vi "Caps_GUI.vi"(11 "GUI_cluster":T1={"Sub Panel"=refnum, "GUIdevice"="Bella_LP_Mode", "CtlRef"=refnum, "User Event in"=refnum}) -> ()   [LabVIEW 2013]
uses:
  Shared/GUI_Template/GUI_master/tcp_new_data_event.ctl
  Shared/GUI_Template/GUI_master/tcp new data cluster.ctl
  Controls/GUI_cluster.ctl
  Controls/eventtypdef1.ctl
panel:
  out "GUIdevice 6":string="Bella_LP_Mode"
  out "GUIdevice 5":string="Bella_LP_Mode"
  out "GUIdevice 4":string="Bella_LP_Mode"
  out "GUIdevice 3":string="Bella_LP_Mode"
  out "GUIdevice 2":string="Bella_LP_Mode"
  out "timing (ns) 2":dbl
  in  "timing (ns)":dbl
  out "pressureCap1::6":dbl caption="pressure read" min=0.0 max=10.0
  out "pressureCap2::6":dbl caption="pressure read" min=0.0 max=10.0
  in  "pressure::5":dbl caption="pressure" min=0.0 max=200.0
  in  "pressure::4":dbl caption="pressure" min=0.0 max=200.0
  in  "discharge2::3":bool caption="Trigger"
  in  "discharge1::3":bool caption="Trigger"
  out "AI_mean.Channel 3::2":dbl caption="read \nvoltage" min=0.0 max=0.0
  in  "voltage.hv 2::1":dbl caption="set \nvoltage" min=0.0 max=30.0
  out "AI_mean.Channel 0::2":dbl caption="read \nvoltage" min=0.0 max=0.0
  in  "voltage.hv 1::1":dbl caption="set \nvoltage" min=0.0 max=30.0
  out "tcp data event":T2
  out "GUIdevice 1":string="Bella_LP_Mode"
  in  "stop":bool
  # "CAP2"
  # "CAP1"
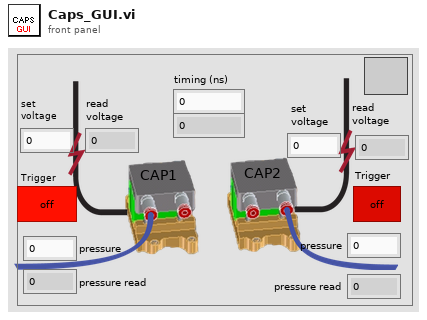
[diagram p1: front panel]
types:
  T1 = typedef "GUI_cluster.ctl" = cluster{"Sub Panel":refnum<vi>, "GUIdevice":string, "CtlRef":refnum<vi>, "User Event in":refnum<user-event>}
  T2 = typedef "tcp_new_data_event.ctl" = refnum<user-event>
  T3 = typedef "eventtypdef1.ctl" = cluster{"label":string, "Sub Panel":refnum<vi>, "CtlRef":refnum<vi>, "This VI":refnum<vi>}
  T4 = typedef "tcp new data cluster.ctl" = cluster{"EventEnum":enum16{"new data", "connection status update"}, "Device name":string}
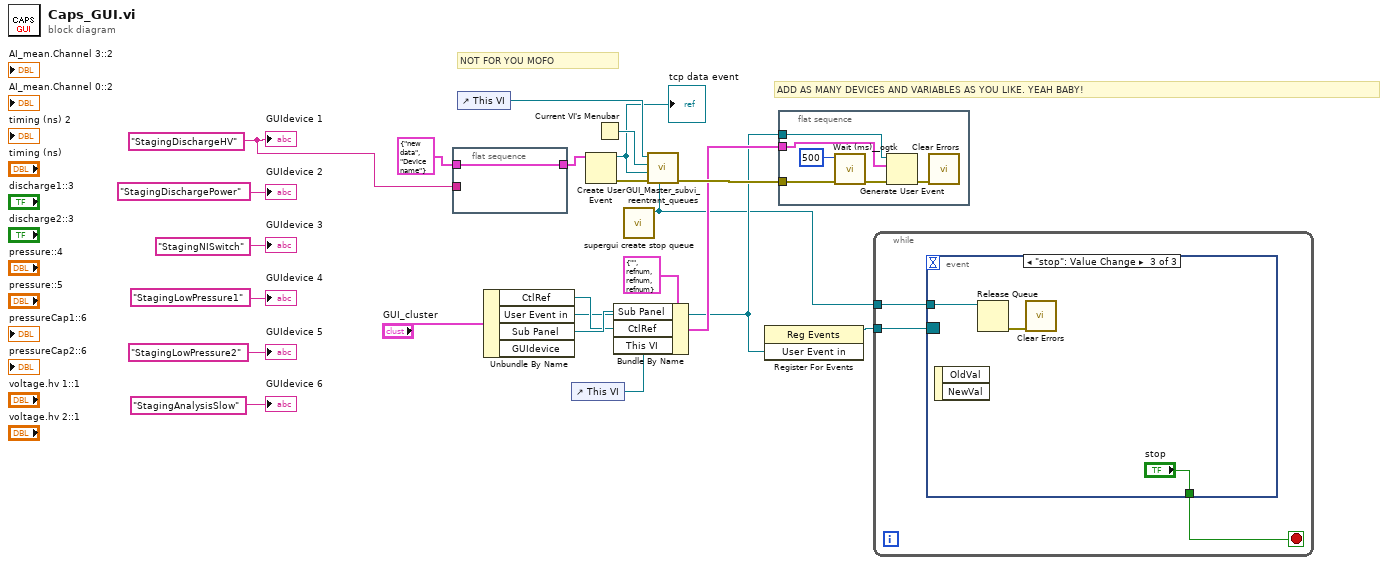
[diagram p0: block diagram]
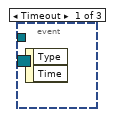
[diagram p2: hidden frame]
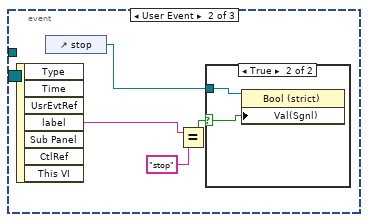
[diagram p3: hidden frame]
diagram:
  w2 = "StagingDischargeHV" ("GUIdevice 23")
  # "ADD AS MANY DEVICES AND VARIABLES AS YOU LIKE. YEAH BABY!"
  # "NOT FOR YOU MOFO"
  n1 = flat-sequence {
    tunnel: T4 {"EventEnum"=enum."new data", "Device name"="Device name"} ("New Event") -> [w23]
    tunnel: w2 -> [_]
    tunnel: [w23] -> w1
    frame #0 {
    }
  }
  n2 = control-ref of="This VI"() -> (w22:refnum<vi>)
  n3 = Unbundle By Name("GUI_cluster") -> ("CtlRef"=w15:refnum<vi>, "User Event in"=w5:refnum<user-event>, "Sub Panel"=w16:refnum<vi>)  [unwired: 1 out]
  n4 = control-ref of="This VI"() -> (w14:refnum<vi>)
  n5 = Create User Event(user event datatype=w1) -> (user event=w19:refnum<user-event>, error out=w20:errorcluster)  [unwired: 1 in]
  "tcp data event" <- w19
  n6 = Current VI's Menubar() -> (w21:refnum<k9>)
  n7 = Bundle By Name(cluster=T3 {"label"="", "Sub Panel"=refnum, "CtlRef"=refnum, "This VI"=refnum} ("event data"), "Sub Panel"=w16, "CtlRef"=w15, "This VI"=w14) -> (w12:T3)
  n8 = call "supergui create stop queue.vi"() -> ("STOP Queue out"=w4:refnum<queue>)  [unwired: 11 in]
  n9 = call "GUI_Master_subvi_reentrant_queues.vi"("STOP Queue in"=w4, "error in (no error)"=w20, "tcp data event"=w19, "Caller menu reference"=w21, "Caller VI ref"=w22) -> ("error out"=w13:errorcluster)  [unwired: 6 in]
  n10 = register-events(w5) -> (reference out=w6:refnum<event-registration>)  [unwired: 2 in, 1 out]
  n11 = flat-sequence {
    tunnel: w13 -> [w26]
    tunnel: w5 -> [w29]
    tunnel: w12 -> [w28]
    frame #0 {
      n12 = call <userlib>:"Wait (ms)__ogtk.vi"("error in (no error)"=w26, "milliseconds to wait"=u32 500) -> ("error out"=w25:errorcluster)  [unwired: 8 in, 1 out]
      n13 = Generate User Event(user event=w29, event data cluster=w28, error in=w25) -> (error out=w27:errorcluster)  [unwired: 1 in, 1 out]
      n14 = call <vilib>:"Clear Errors.vi"("error in (no error)"=w27) -> ()  [unwired: 6 in, 1 out]
    }
  }
  n15 = while {
    tunnel: w6 -> [w32]
    tunnel: w4 -> [w30]
    stop <- w31 stop-if-true
    n16 = event shown="[2] \"stop\": Value Change" {
      selector: w32 -> [_ _ _]
      dyn-events: _ -> [_ _ _]
      timeout: _ -> [_ _ _]
      tunnel: [_ _ "stop"] -> w31
      tunnel: w30 -> [_ _ w40]
      event Timeout {
        n17 = event-data() -> ()  [unwired: 1 in, 2 out]
      }
      event User Event {
        n18 = event-data() -> ("label"=w36:string)  [unwired: 1 in, 6 out]
        n19 = control-ref of="stop"() -> (w33:refnum<vi>)
        n20 = Equal?(x=w36, y="stop") -> (x = y?=w34:bool)
        n21 = case shown="True" w34 {
          selector: w34 -> [_ w37]
          tunnel: w33 -> [_ w38]
          frame False {
          }
          frame True {
            n22 = property class="Bool (strict)"(reference=w38, "Val(Sgnl)"=w37) -> ()  [unwired: 1 in, 2 out]
          }
        }
      }
      event "stop": Value Change {
        n23 = event-data() -> ()  [unwired: 1 in, 2 out]
        n24 = Release Queue(queue=w40) -> (error out=w39:errorcluster)  [unwired: 2 in, 2 out]
        n25 = call <vilib>:"Clear Errors.vi"("error in (no error)"=w39) -> ()  [unwired: 6 in, 1 out]
      }
    }
  }
  "GUIdevice 1" <- w2
  "GUIdevice 2" <- "StagingDischargePower" ("GUIdevice 23")
  "GUIdevice 3" <- "StagingNISwitch" ("GUIdevice 8")
  "GUIdevice 4" <- "StagingLowPressure1" ("GUIdevice 2")
  "GUIdevice 5" <- "StagingLowPressure2" ("GUIdevice 2")
  "GUIdevice 6" <- "StagingAnalysisSlow" ("GUIdevice 1")
